vi "查看未注册设备.vi"(10 "要查询的企业":string[](array[string]), 11 "数据库连接引用.i":T1) -> (2 "所有未注册设备":cluster{"企业数据库名":string, "未注册设备":string[]}[](array[cluster]), 3 "数据库连接引用.o":T1)   [LabVIEW 2013, in "数据库操作.lvclass"]
uses:
  <vilib>/addons/database/Connection.llb/Conn ObjectReference.ctl
  <vilib>/addons/database/Connection.llb/Conn Execute.vi
  <vilib>/addons/database/NI_Database_API.lvlib
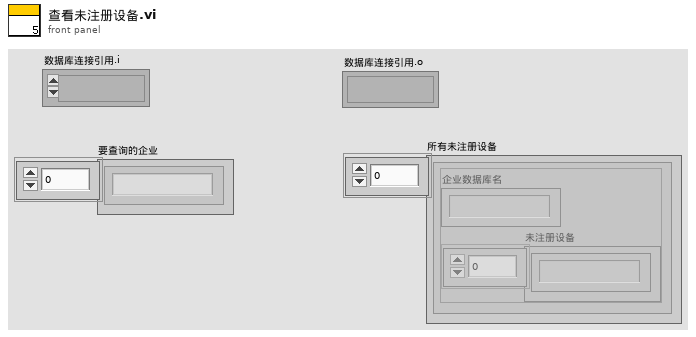
[diagram p1: front panel]
types:
  T1 = typedef "NI_Database_API.lvlib/Conn ObjectReference.ctl" = refnum<k1>
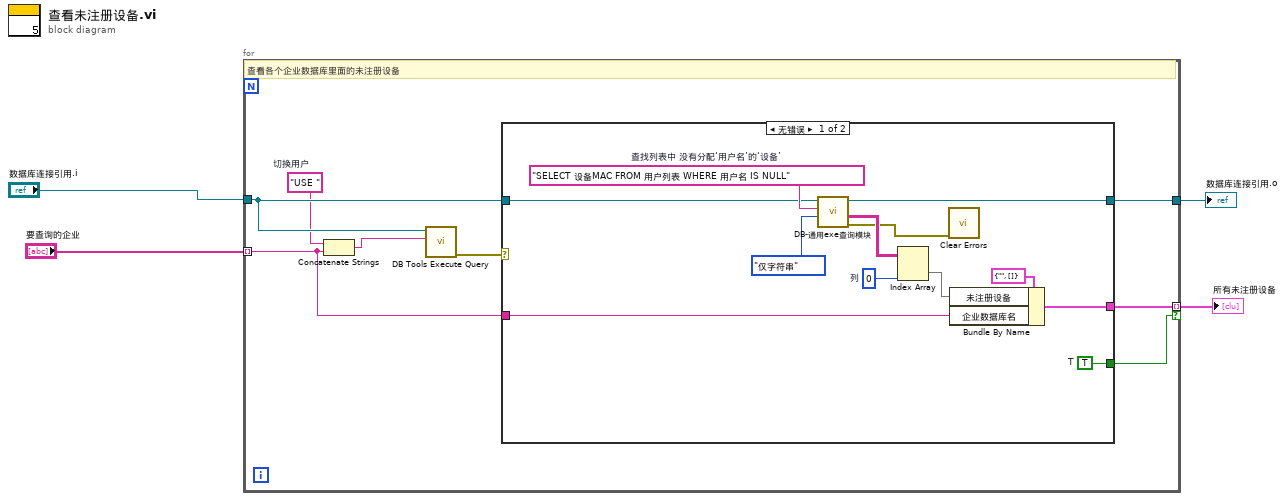
[diagram p0: block diagram]
diagram:
  n1 = for {
    tunnel: "数据库连接引用.i" -> [w12]
    tunnel: "要查询的企业" -> [w7] mode=indexing
    tunnel: [w6] -> w3 mode=indexing if=w8
    tunnel: [w5] -> w1
    w11 = "USE "  # 切换用户
    # "查看各个企业数据库里面的未注册设备"
    n2 = Concatenate Strings(w11, w7) -> (w10:string)
    n3 = call-poly <vilib>:"DB Tools Execute Query.vi"("SQL query"=w10, "connection reference"=w12) -> ("error out"=w9:errorcluster)  [unwired: 6 in, 1 out]
    n4 = case shown="无错误" w9 {
      tunnel: w12 -> [w19 w25]
      tunnel: [w18 _] -> w8
      tunnel: w7 -> [w16 _]
      tunnel: [w14 _] -> w6
      tunnel: [w13 w25] -> w5
      frame No Error {
        w18 = TRUE  # T
        w21 = 0  # 列
        w24 = "SELECT 设备MAC FROM 用户列表 WHERE 用户名 IS NULL"  # 查找列表中 没有分配‘用户名’的‘设备’
        n5 = call "DB-通用exe查询模块.vi"("解析模式"=enum16{"仅数值", "仅字符串", "数值与字符串"}."仅字符串", "SQL query"=w24, "数据库连接引用"=w19) -> ("error out"=w20:errorcluster, "字符串数据"=w22:string[][], "数据库连接引用out"=w13:T1)  [unwired: 5 in, 1 out]
        n6 = Index Array(array=w22, index (col)=w21) -> (element=w15:string[])  [unwired: 1 in]
        n7 = call <vilib>:"Clear Errors.vi"("error in (no error)"=w20) -> ()  [unwired: 6 in, 1 out]
        n8 = Bundle By Name(cluster=cluster{"企业数据库名":string, "未注册设备":string[]} {"企业数据库名"="", "未注册设备"=[]}, "未注册设备"=w15, "企业数据库名"=w16) -> (w14:cluster{"企业数据库名":string, "未注册设备":string[]})
      }
      frame Error {
      }
    }
  }
  "所有未注册设备" <- w3
  "数据库连接引用.o" <- w1
